vi "Error Log.vi"(8 "error in (no error)":errorcluster, 11 "Object in":refnum<class>) -> (0 "error out":errorcluster)   [LabVIEW 2026, in "TALOS.lvlib"]
uses:
  TALOS.lvlib
  Ancestor/Ancestor/Ancestor.lvclass/Ancestor.ctl
  FGV/Error Memory/Get Error Description.vi
  Get PC name.vi
  Ancestor/Ancestor/Read ID.vi
  Get Class Name.vi
  <vilib>/Utility/error.llb/Clear Errors.vi
  FGV/Error Memory/Error Memory Core.vi
  <vilib>/AdvancedString/Delimited String to 1D String Array.vi
  <vilib>/AdvancedString/Delimited String to 1D String Array (string).vi
  Circus Root Path.vi
  FGV/Error Memory/Error Crt Lvl checker.vi
  FGV/Error Memory/Error Memory Core.vi/40c8088d-b597-4017-91af-faa98e00292e.vi
  FGV/Error Memory/Error Memory Core.vi/d4a3ab98-063c-4e44-b43d-fbdcfe6c2be2.vi
  Global Memory.vi
  <vilib>/Utility/LVClass/Get LV Class Name.vi
  Is in Packed Library.vi
  TALOS Root path.vi
  Read CSV worksheet.vi
  Global Constants.vi
  <vilib>/Utility/error.llb/General Error Handler.vi
  <vilib>/Utility/config.llb/Open Config Data.vi
  <vilib>/Utility/config.llb/Get Section Names.vi
  <vilib>/Utility/config.llb/Get Key Names.vi
  <vilib>/Utility/config.llb/Read Key.vi
  <vilib>/Utility/config.llb/Read Key (String).vi
  <vilib>/Utility/config.llb/Close Config Data.vi
  Ancestor/Ancestor/Ancestor.lvclass
  <vilib>/Comparison/Equal/Equal Functor/Equal Functor.lvclass
  Classes/Log/Log.lvclass
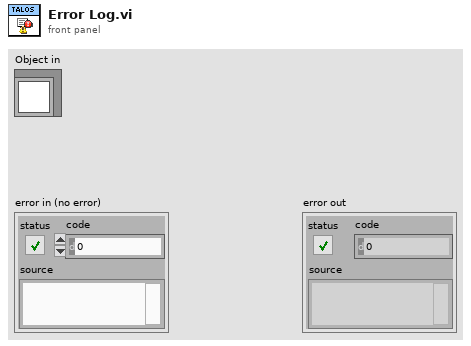
[diagram p1: front panel]
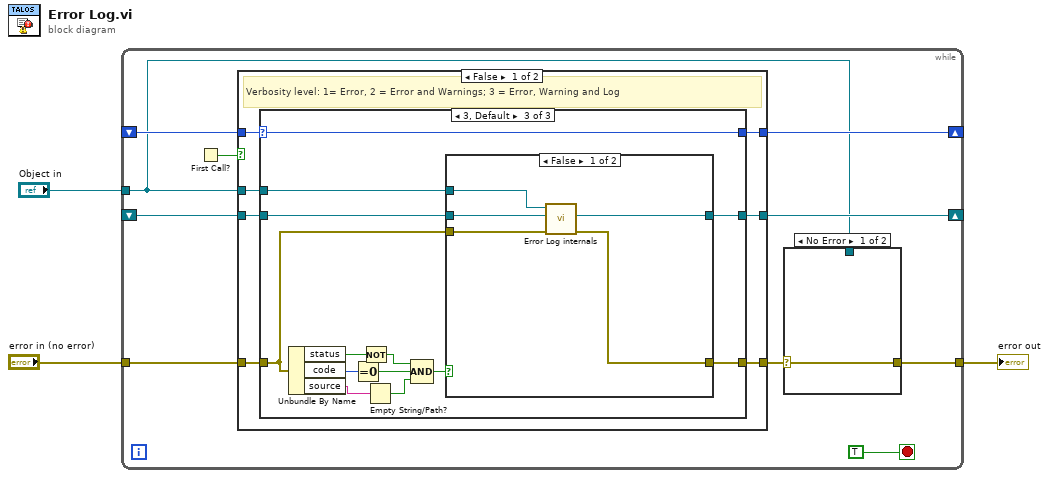
[diagram p0: block diagram]
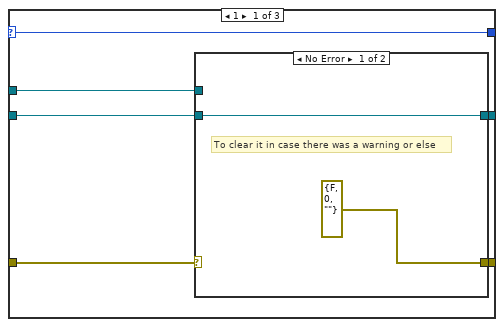
[diagram p2: hidden frame]
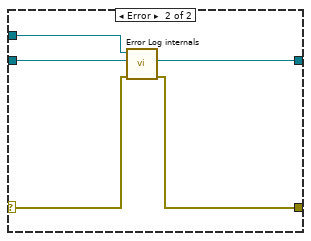
[diagram p3: hidden frame]
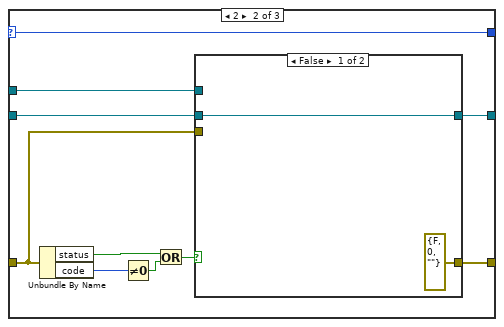
[diagram p4: hidden frame]
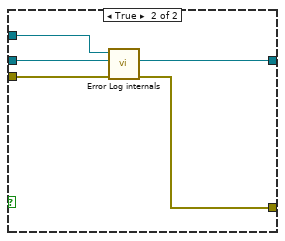
[diagram p5: hidden frame]
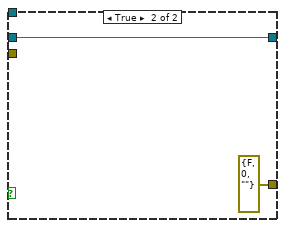
[diagram p6: hidden frame]
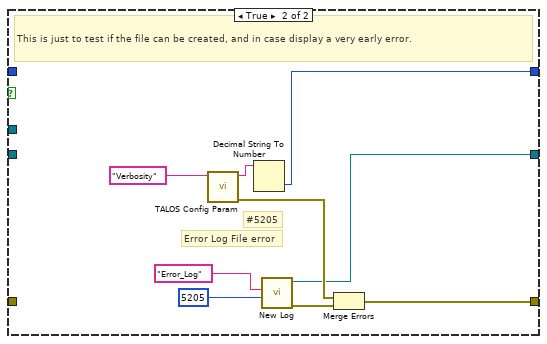
[diagram p7: hidden frame]
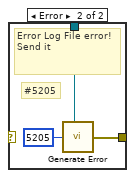
[diagram p8: hidden frame]
diagram:
  n1 = while {
    shift-right: [w11] -> _
    shift-left: _ -> [w10]
    tunnel: "Object in" -> [w6]
    shift-right: [w9] -> _
    shift-left: _ -> [w8]
    tunnel: [w4] -> w3
    tunnel: "error in (no error)" -> [w5]
    stop <- TRUE stop-if-true
    n2 = First Call?() -> (First Call?: T/F=w12:bool)
    n3 = case shown="False" w12 {
      tunnel: [w19 w72] -> w11
      tunnel: w10 -> [w20 _]
      tunnel: w6 -> [w18 _]
      tunnel: [w15 w76] -> w9
      tunnel: w8 -> [w16 _]
      tunnel: w5 -> [w17 _]
      tunnel: [w14 w75] -> w7
      frame False {
        # "Verbosity level: 1= Error, 2 = Error and Warnings; 3 = Error, Warning and Log"
        n4 = case shown="3, Default" w16 {
          selector: w16 -> [w23 w36 w60]
          tunnel: w20 -> [w26 w43 w63]
          tunnel: [w25 w42 w62] -> w19
          tunnel: w18 -> [w24 w41 w61]
          tunnel: w17 -> [w21 w34 w58]
          tunnel: [w23 w36 w60] -> w15
          tunnel: [w22 w35 w59] -> w14
          frame 1 {
            n5 = case shown="No Error" w21 {
              selector: w21 -> [_ w32]
              tunnel: w26 -> [w28 w33]
              tunnel: [w28 w29] -> w25
              tunnel: w24 -> [_ w31]
              tunnel: [errorcluster {"status"=FALSE, "code"=0, "source"=""} ("error out") w30] -> w22
              frame No Error {
                # "To clear it in case there was a warning or else"
              }
              frame Error {
                n6 = call "Error Log internals.vi"("error in (no error)"=w32, "Log in"=w33, "Object in"=w31) -> ("error out"=w30:errorcluster, "Log out"=w29:refnum<class "Log.lvclass">)  [unwired: 7 in]
              }
            }
          }
          frame 2 {
            n7 = Unbundle By Name(w34) -> ("status"=w40:bool, "code"=w39:i32)
            n8 = Not Equal To 0?(x=w39) -> (x != 0?=w38:bool)
            n9 = Or(x=w40, y=w38) -> (x .or. y?=w37:bool)
            n10 = case shown="False" w37 {
              tunnel: w43 -> [w45 w48]
              tunnel: [w45 w47] -> w42
              tunnel: w41 -> [_ w50]
              tunnel: [errorcluster {"status"=FALSE, "code"=0, "source"=""} ("error out") w49] -> w35
              tunnel: w34 -> [_ w46]
              frame False {
              }
              frame True {
                n11 = call "Error Log internals.vi"("error in (no error)"=w46, "Log in"=w48, "Object in"=w50) -> ("error out"=w49:errorcluster, "Log out"=w47:refnum<class "Log.lvclass">)  [unwired: 7 in]
              }
            }
          }
          frame 3, Default {
            n12 = Unbundle By Name(w58) -> ("status"=w56:bool, "code"=w57:i32, "source"=w53:string)
            n13 = Equal To 0?(x=w57) -> (x = 0?=w54:bool)
            n14 = Not(x=w56) -> (.not. x?=w55:bool)
            n15 = Empty String/Path?(string/path=w53) -> (empty?=w52:bool)
            n16 = Compound Arithmetic op=AND(w55, w54, w52) -> (w51:bool)
            n17 = case shown="False" w51 {
              tunnel: w63 -> [w66 w70]
              tunnel: [w65 w70] -> w62
              tunnel: w61 -> [w68 _]
              tunnel: [w67 errorcluster {"status"=FALSE, "code"=0, "source"=""} ("error out")] -> w59
              tunnel: w58 -> [w64 _]
              frame False {
                n18 = call "Error Log internals.vi"("error in (no error)"=w64, "Log in"=w66, "Object in"=w68) -> ("error out"=w67:errorcluster, "Log out"=w65:refnum<class "Log.lvclass">)  [unwired: 7 in]
              }
              frame True {
              }
            }
          }
        }
      }
      frame True {
        # "Error Log File error"
        # "#5205"
        # "This is just to test if the file can be created, and in case display a very early error."
        n19 = call "TALOS Config Param.vi"("Parameter Name"="Verbosity") -> ("error out"=w78:errorcluster, "Output"=w77:string)  [unwired: 9 in]
        n20 = Decimal String To Number(string=w77) -> (number=w76:i32)  [unwired: 2 in, 1 out]
        n21 = call "New Log.vi"("Specific Error Code"=5205 ("Error Code"), "Name"="Error_Log") -> ("error out"=w71:errorcluster, "Log out"=w72:refnum<class "Log.lvclass">)  [unwired: 8 in]
        n22 = Merge Errors(w78, w71) -> (w75:errorcluster)
      }
    }
    n23 = case shown="No Error" w7 {
      selector: w7 -> [w80 _]
      tunnel: [w80 w82] -> w4
      tunnel: w6 -> [_ w81]
      frame No Error {
      }
      frame Error {
        # "#5205"
        # "Error Log File error! Send it"
        n24 = call "Generate Error.vi"("Class"=w81, "Error Code"=5205) -> ("error out"=w82:errorcluster)  [unwired: 5 in]
      }
    }
  }
  "error out" <- w3
